vi "All on test.vi"(7 "system state in in":T2, 11 "mode set":T1) -> (8 "system state out":T2)   [LabVIEW 2016]
doc: "This subvi just keeps all the lights in the 4 way intersection on until is told not to do so.\n\nAlexis Lopez\nP350\nCUSUB Physics"
uses:
  typedefs/system state cluster.ctl
  typedefs/state enum.ctl
  typedefs/control mode enum.ctl
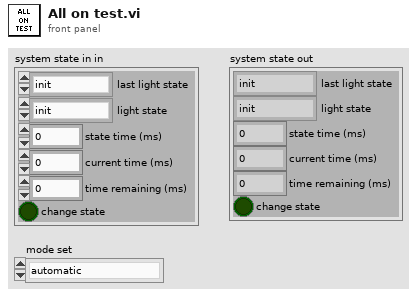
[diagram p1: front panel]
types:
  T1 = typedef "control mode enum.ctl" = enum16{"automatic", "blinking", "all on test"}
  T2 = typedef "system state cluster.ctl" = cluster{"last light state":T3, "light state":T3, "state time (ms)":i32, "current time (ms)":i32, "time remaining (ms)":i32, "change state":bool}
  T3 = typedef "state enum.ctl" = enum16{"init", "idle", "left turn E", "go EW", "caution EW", "left turn W", "left turn N", "go NS", "caution NS", "left turn S", "blink on", "blink off", "all on test", "exit"}
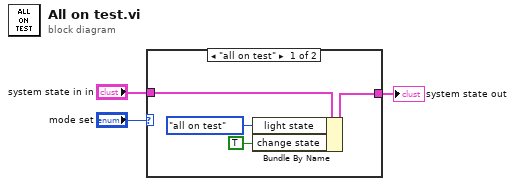
[diagram p0: block diagram]
diagram:
  n1 = case shown="\"all on test\"" "mode set" {
    tunnel: "system state in in" -> [w7 w8]
    tunnel: [w6 w8] -> w2
    frame "all on test" {
      n2 = Bundle By Name(cluster=w7, "light state"=state_enum."all on test", "change state"=TRUE) -> (w6:T2)
    }
    frame "blinking", Default {
    }
  }
  "system state out" <- w2
